vi "Dashboard Main.vi"() -> ()   [LabVIEW 2016]
uses:
  <vilib>/Utility/miscctls.llb/LVRowAndColumnTypeDef.ctl
  <vilib>/event_ctls.llb/eventvkey.ctl
  <vilib>/Rock Robotics/Network Tables/NT Read Numeric Array.vi
  <vilib>/Rock Robotics/Network Tables/NT Read Boolean.vi
  <vilib>/Rock Robotics/WPI/Dashboard/WPI_DashboardLogging Global.vi
  <vilib>/Math Plots/2D Math Plots/2D Compass/2D Compass Datatype/Public/Plot Helper (Vector).vi
  <vilib>/Math Plots/2D Math Plots/2D Compass/2D Compass Datatype/2D Compass Datatype.lvclass
panel:
  in  "Camera Settings Right":T1={"Frame Rate"=30, "Compression"=30, "Size"=1, "DB Camera Config"=FALSE} {"Frame Rate" scale=1.0..30.0; "Compression" scale=100.0..-1.0; "Size" items=["640x480", "320x240", "160x120"]}
  in  "Camera Name Right":string(combo)="No Camera Selection"
  out "Camera Info":cluster{"Mbps LED":bool, "Mbps":dbl, "fps":dbl} {"fps" format="%#.1g"; "Mbps" format="%#.1g"}
  in  "Camera Settings":T1={"Frame Rate"=30, "Compression"=30, "Size"=1, "DB Camera Config"=FALSE} {"Frame Rate" scale=1.0..30.0; "Compression" scale=100.0..-1.0; "Size" items=["640x480", "320x240", "160x120"]}
  in  "TCP":refnum<k5>
  in  "Rec Mode":enum32{"Stop", "Record", "Playback"}(radio)
  out "Robot IP":string
  out "Image Message":string="Timeout in Camera Communications"
  in  "Dashboard Tab":T2(tab)
  in  "Select Auto":string(combo)="Select Autonomous ..."
  out "NT Connection":bool
  out "MotorChart R":cluster{"Numeric":dbl, "Numeric":dbl}(graph)
  out "MotorChart L":cluster{"Numeric":dbl, "Numeric":dbl}(graph)
  out "MotorSliders R":cluster{"MotorSlide1":dbl, "MotorSlide2":dbl} {"MotorSlide2" scale=-1.0..1.0 scale format="%#_2e"; "MotorSlide1" scale=-1.0..1.0 scale format="%#_2e"}
  out "MotorSliders L":cluster{"MotorSlide1":dbl, "MotorSlide2":dbl} {"MotorSlide2" scale=-1.0..1.0 scale format="%#_2e"; "MotorSlide1" scale=-1.0..1.0 scale format="%#_2e"}
  out "Gyro":dbl(knob) scale=0.0..360.0
  out "JS1 Z":dbl(slide) scale=-1.0..1.0 scale format="%#_2e"
  out "JS1 Graph":cluster{"X":dbl, "Y":dbl}[](graph)
  out "JS1 Buttons":T3
  out "JS2 Z":dbl(slide) scale=-1.0..1.0 scale format="%#_2e"
  out "JS2 Graph":cluster{"X":dbl, "Y":dbl}[](graph)
  out "JS2 Buttons":T3
  out "Mode":T4(ring)=enum."Auto Disabled"
  out "Camera Image Right":T5(plugin-control)
  in  "DB/String 9":string
  in  "DB/String 8":string
  in  "DB/String 7":string
  in  "DB/String 6":string
  in  "DB/String 5":string
  in  "DB/String 4":string
  in  "DB/String 3":string
  in  "DB/String 2":string
  in  "DB/String 1":string
  in  "DB/String 0":string
  in  "DB/Slider 0":dbl(slide) scale=0.0..5.0
  in  "DB/Slider 1":dbl(slide) scale=0.0..5.0
  in  "DB/Slider 2":dbl(slide) scale=0.0..5.0
  in  "DB/Slider 3":dbl(slide) scale=0.0..5.0
  out "DB/LED 3":bool
  out "DB/LED 2":bool
  out "DB/LED 1":bool
  out "DB/LED 0":bool
  in  "DB/Button 3":bool
  in  "DB/Button 2":bool
  in  "DB/Button 1":bool
  in  "DB/Button 0":bool caption="New Name"
  out "Position Z":dbl
  out "Position Y":dbl
  out "Position X":dbl
  out "Velocity Z":dbl
  out "Velocity Y":dbl
  out "Velocity X":dbl
  in  "Auto Select":dbl
  out "Horizontal Heading":u8(slide) scale=0.0..100.0
  out "Vertical Heading":u8(slide) scale=0.0..100.0
  out "Slow":bool
  out "Fast":bool
  out "Reversed":bool
  out "Right Speed":dbl(knob) scale=0.0..1.0
  out "Left Speed":dbl(knob) scale=0.0..1.0
  out "Right Encoder":dbl
  out "Left Encoder":dbl
  in  "Test Slider":dbl(slide) scale=0.0..100.0 scale format="%#_3g"
  in  "On/Off":bool caption="Solenoid"
  in  "Test Name":u16(ring) items=["Select the test to run..."]
  in  "Test Tree":string(tree)
  in  "Motor":cluster{"Value":dbl, "Enable":bool} {"Value" scale=-1.0..1.0 scale format="%#_3g"}
  out "Progress":T6 {"Test Progress" scale=0.0..100.0}
  in  "Rev/Fwd":cluster{"Forward":bool, "Reverse":bool}
  in  "Test Ring":u16(ring) items=["Monochrome", "Color"]
  out "Cmd Status":string
  in  "Execute Command":bool
  in  "Command Params":string[][](table)
  in  "Command Selection":i32(listbox)
  in  "CheckList":i32(listbox)
  out "Tree":string(tree)
  out "Camera Image":T5(plugin-control)
  out "Background":bool
  in  "Camera Name":string(combo)="No Camera Selection"
  # "HW"
  # "HW"
  # "Joysticks"
  # "Drive Motors"
  # "Front"
  # "Right"
  # "Left"
  # "Back"
  # "1. Center Auto\n2. Left Auto\n3. Right Auto\n\n** Defaults to 1"
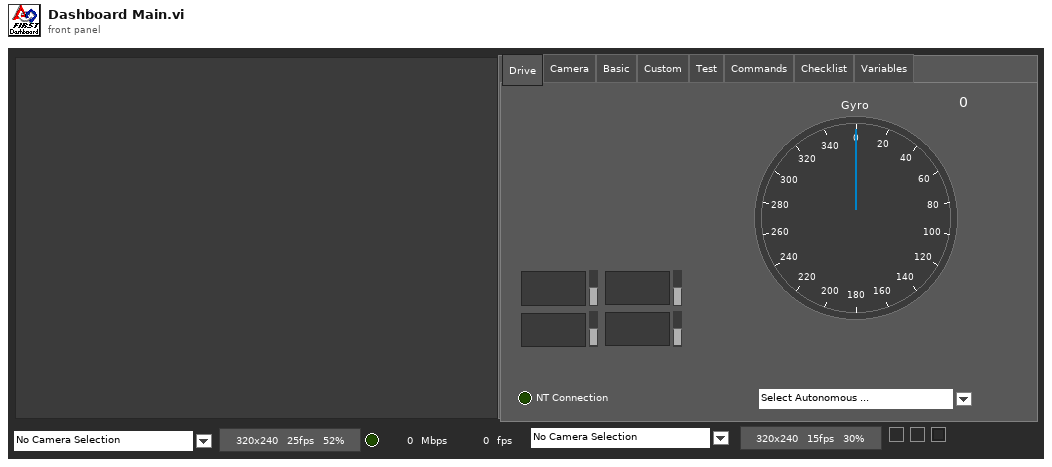
[diagram p1: front panel]
types:
  T1 = cluster{"Frame Rate":i32, "Compression":i32, "Size":u16, "DB Camera Config":bool}
  T2 = enum32{"Drive", "Camera", "Basic", "Custom", "Test", "Commands", "Checklist", "Variables"}
  T3 = cluster{bool, bool, bool, bool, bool, bool, bool, bool, bool, bool, bool, bool}
  T4 = enum8{"Tele-Op Disabled", "Tele-Op Enabled", "Auto Disabled", "Auto Enabled", "Test Disabled", "Test Enabled", "Disconnected", "No Code", "E-Stop"}
  T5 = typedef "IMAQ Image.ctl" = refnum<image>
  T6 = cluster{"Test Progress":u8, "Test Progress Text":string}
  T7 = typedef "Image Type" = u32
  T8 = cluster{"IDs":cluster{"RPC field ID":u16, "Unique ID":u16}, "String":string}
  T9 = enum32{"Drive", "Basic", "Custom", "Test", "Checklist", "Variables"}
  T10 = cluster{"Error Strings":string, "Disable Counts":cluster{u16, u16}, "Rail Faults":cluster{u16, u16, u16}, "Robot IP":string, "DB Mode":u8, "Event Info":cluster{"Name":string, "Type":u8, "Number":u16, "Replay":u8}}
  T11 = cluster{"Storage":cluster{"Disk Free":u64, "RAM Block":u32, "RAM free":u32}, "CPU Utilization":cluster{"CPU % ISR":sgl, "CPU % Time Crit":sgl, "CPU % Timed Str":sgl, "CPU % High":sgl, "CPU % Above":sgl, "CPU % Normal":sgl, "CPU % Low":sgl}, "CAN":cluster{"% Bus Utilization":sgl, "Bus Off Cnt":u32, "TX_FIFO Full Cnt":u32, "Receive Error Cnt":u8, "Transmit Error Cnt":u8}, "HID":cluster{"HID Outputs":u32, "Rumble Low":u16, "Rumble High":u16}[]}
  T12 = cluster{"Status bits":cluster{"Test Mode":bool, "Autonomous":bool, "Enabled":bool, "Code Start":bool, "Brownout":bool, "Reserved 2":bool, "Reserved 3":bool, "E-Stop":bool}, "Code Trace":cluster{"Disabled":bool, "TeleOp":bool, "Auto":bool, "Test":bool}, "Controller Type":enum16{"unknown", "cRIO", "roboRio"}, "Code?":enum16{"unknown", "noCode", "code"}, "Battery V":dbl}
  T13 = cluster{"Control Bits":cluster{"TestMode":bool, "Autonomous":bool, "Enabled":bool, "FMS Present":bool, bool, bool, bool, "E-Stop":bool}, "Team Station ":u8, "Countdown":sgl, "Joystick Values":cluster{"Axes":dbl[], "Buttons":bool[], "POVs":i16[]}[]}
  T14 = cluster{"Axes":dbl[], "Buttons":bool[], "POVs":i16[]}[]
  T15 = cluster{"Axes":dbl[], "Buttons":bool[], "POVs":i16[]}
  T16 = cluster{"Buttons[0]":bool, "Buttons[1]":bool, "Buttons[2]":bool, "Buttons[3]":bool, "Buttons[4]":bool, "Buttons[5]":bool, "Buttons[6]":bool, "Buttons[7]":bool, "Buttons[8]":bool, "Buttons[9]":bool, "Buttons[10]":bool, "Buttons[11]":bool}
  T17 = cluster{"Camera Image":refnum<vi>, "Dashboard Tab":refnum<vi>, "Background":refnum<vi>, "Rec Mode":refnum<vi>, "Test Slider":refnum<vi>, "On/Off ":refnum<vi>, "Test Ring":refnum<vi>, "Rev/Fwd":refnum<vi>, "Test Name":refnum<vi>, "Motor":refnum<vi>, "Progress":refnum<vi>, "CheckList":refnum<vi>, "Tree":refnum<vi>, "Test Tree":refnum<vi>, "Command Params":refnum<vi>, "Command Selection":refnum<vi>, "Execute Command":refnum<vi>, "Cmd Status":refnum<vi>, "Camera Settings":refnum<vi>, "Camera Name":refnum<vi>, "Camera Info":refnum<vi>, "Camera Settings Right":refnum<vi>, "Camera Name Right":refnum<vi>, "Camera Image Right":refnum<vi>}
  T18 = cluster{"Operation":enum16{"Update", "Clear"}, "Color Box":u32}[]
  T19 = typedef "eventvkey.ctl" = enum16{"ASCII", "Enter", "Return", "Shift", "Ctrl", "Alt", "Cmd", "Opt", "Caps", "NumLock", "Clear", "Break", "Up", "Down", "Left", "Right", "Insert", "Delete", "Home", "End", "PageUp", "PageDown", "Escape", "Help", "Pause", "ScrollLock", "F1", "F2", "F3", "F4", "F5", "F6", "F7", "F8", "F9", "F10", "F11", "F12", "F13", "F14", "F15", "F16", "F17", "F18", "F19", "F20", "F21", "F22", "F23", "F24", "Play", "VolumeUp", "VolumeDown", "Mute", "Two Byte Char"}
  T20 = cluster{"Image Size":bool, "Image Type":bool, "Pixel Value":bool, "ROI Information":bool, "Zoom Factor":bool}
  T21 = cluster{"Operation":enum16{"Update", "Clear"}, "Color Box":u32}
  T22 = typedef "LVRowAndColumnTypeDef.ctl" = cluster{"Row":i32, "Column":i32}
  T23 = cluster{"Shift":bool, "Ctrl":bool, "Alt":bool, "Cmd":bool, "Opt":bool}
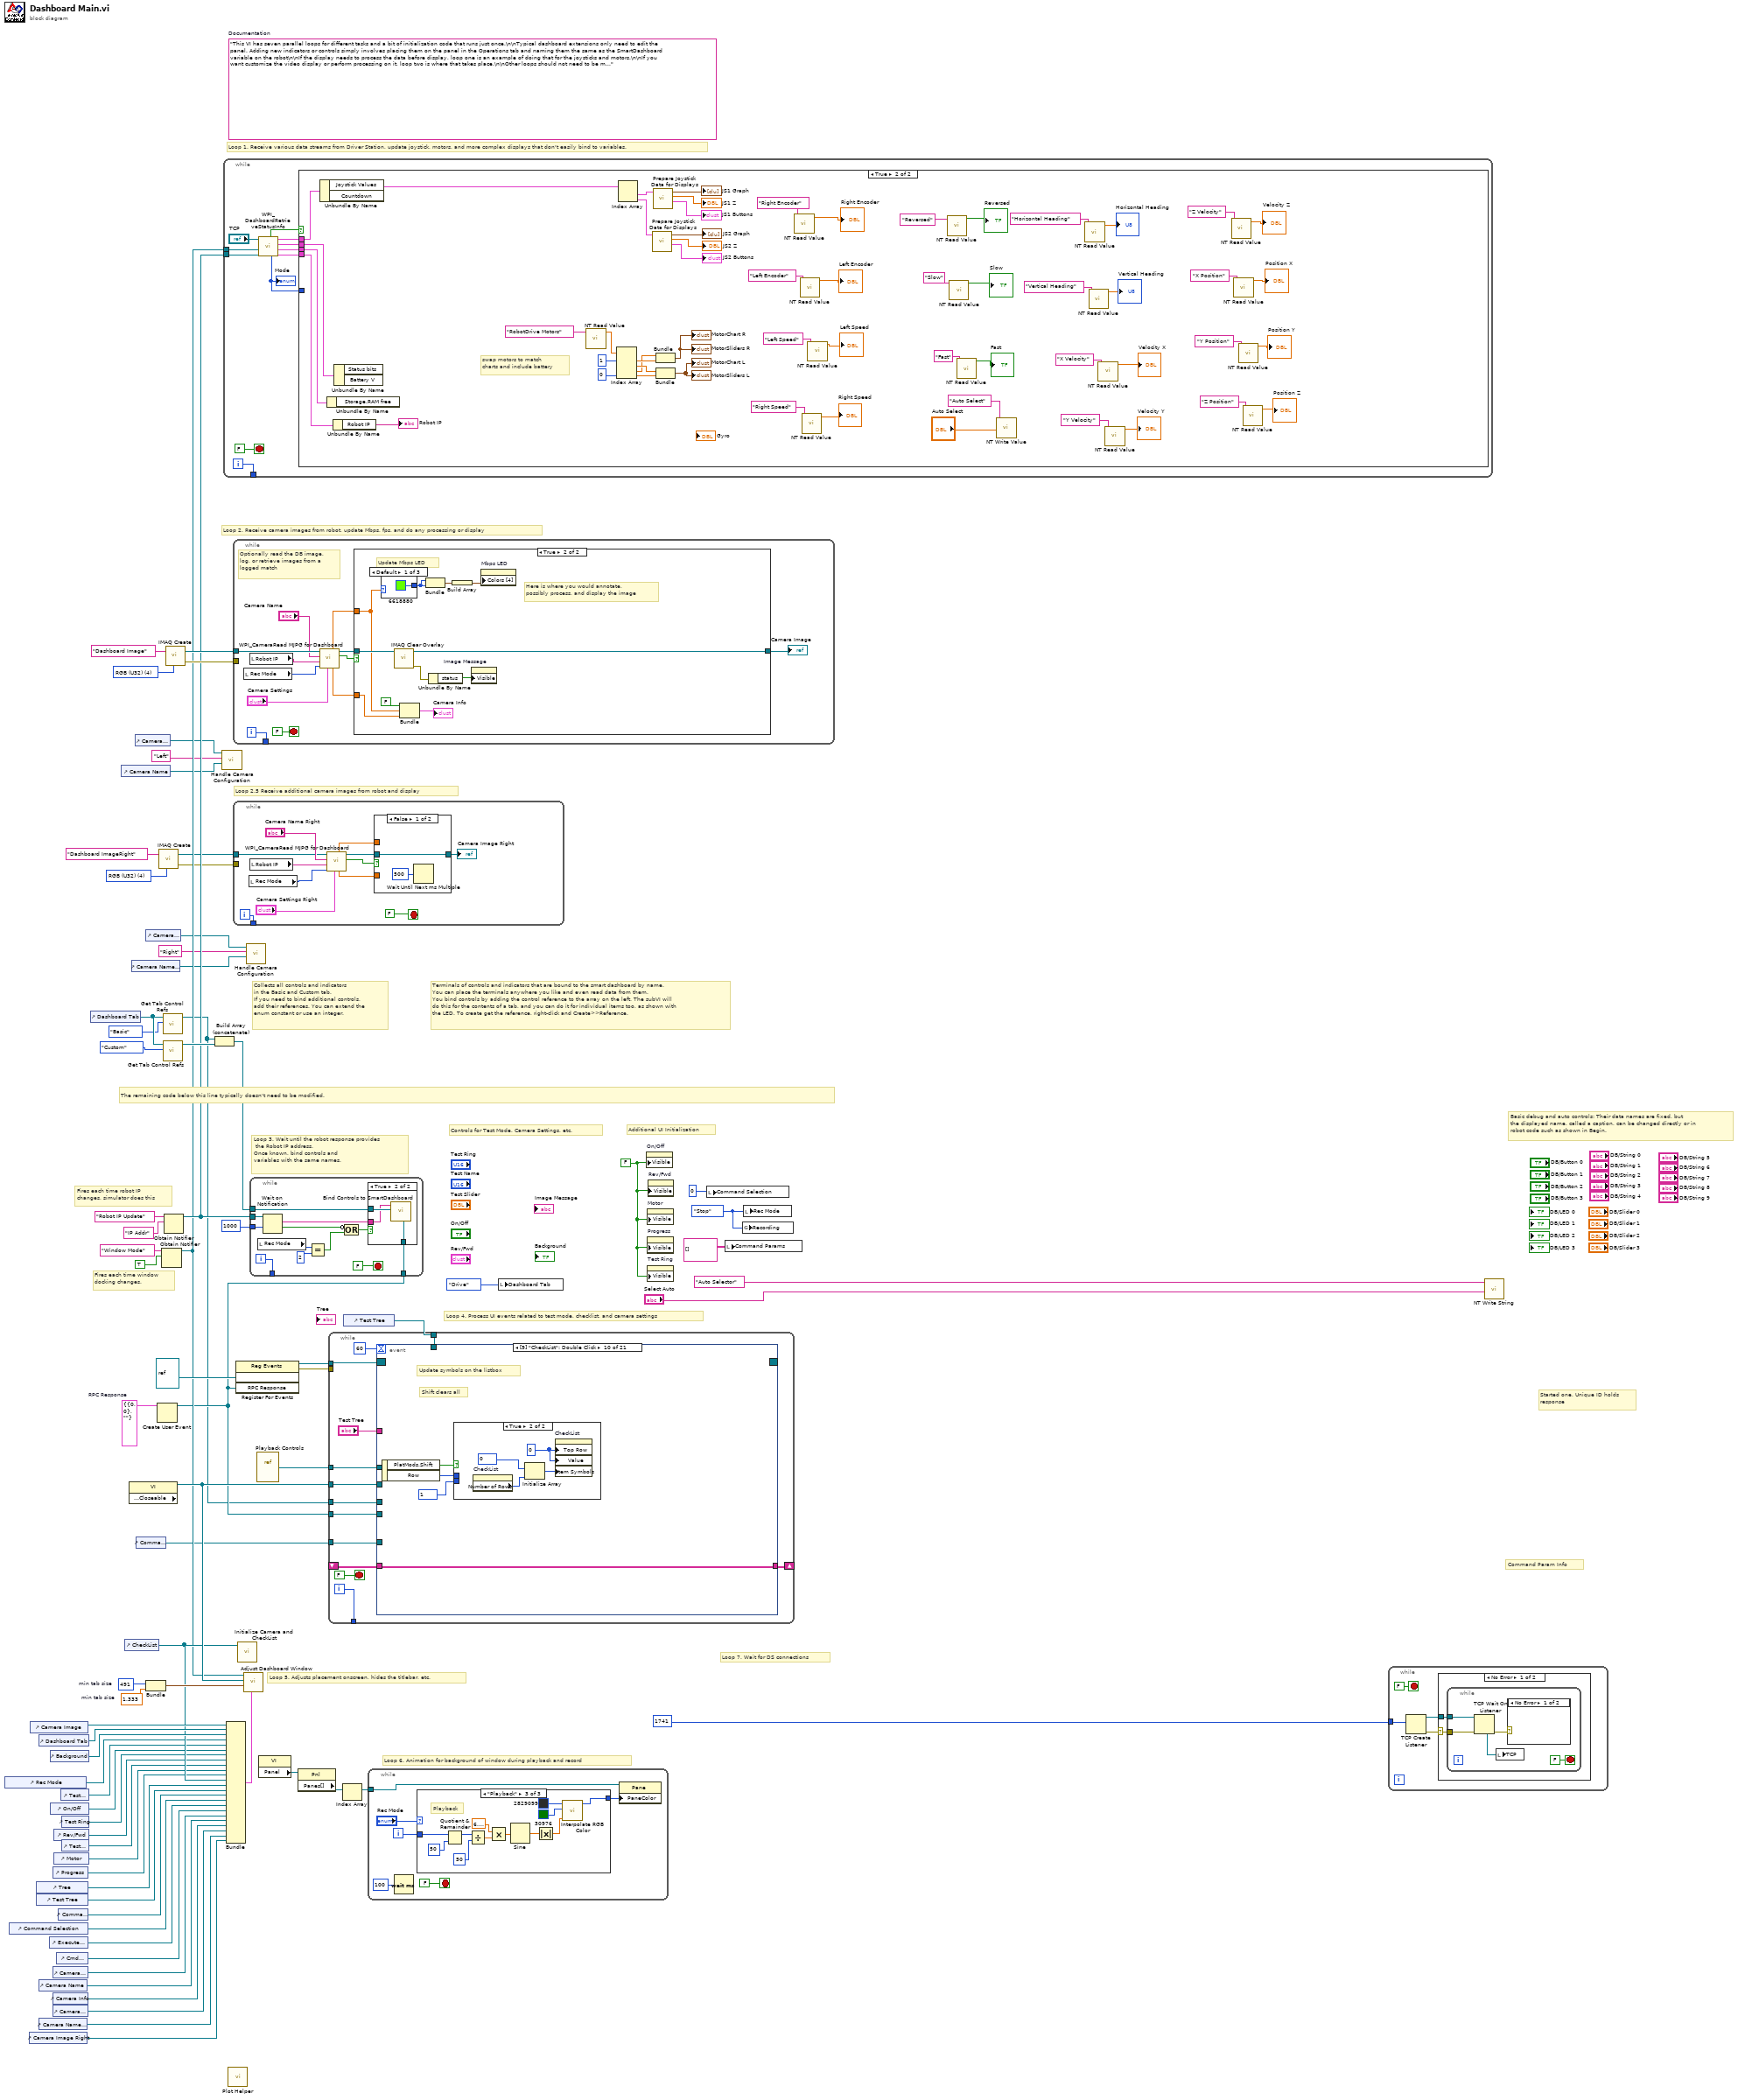
[diagram p0: block diagram]
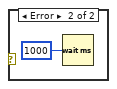
[diagram p3: hidden frame]
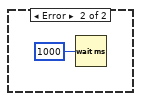
[diagram p4: hidden frame]
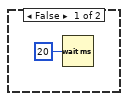
[diagram p5: hidden frame]
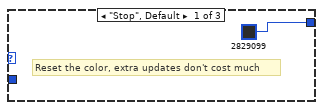
[diagram p6: hidden frame]
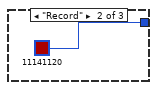
[diagram p7: hidden frame]
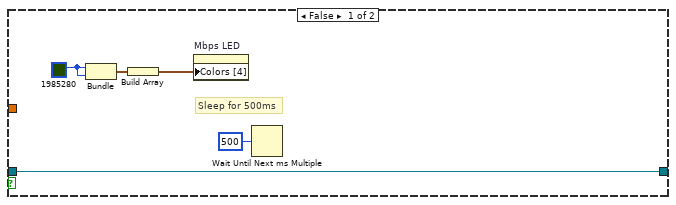
[diagram p9: hidden frame]
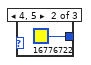
[diagram p10: hidden frame]
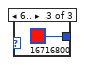
[diagram p11: hidden frame]
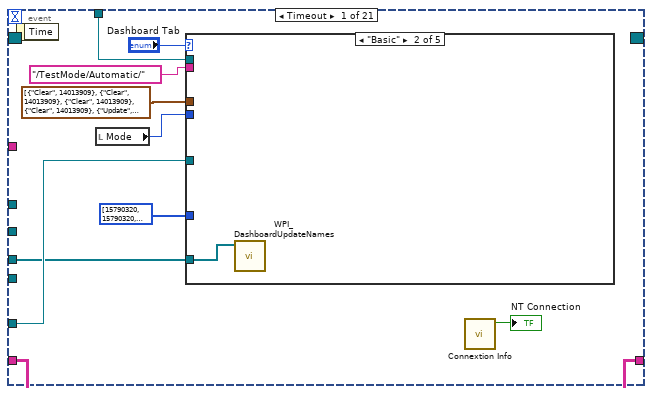
[diagram p12: hidden frame]
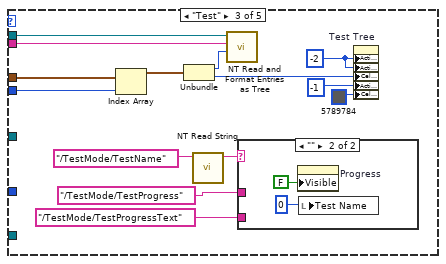
[diagram p14: hidden frame]
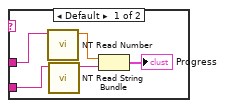
[diagram p15: hidden frame]
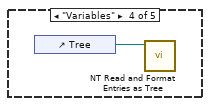
[diagram p16: hidden frame]
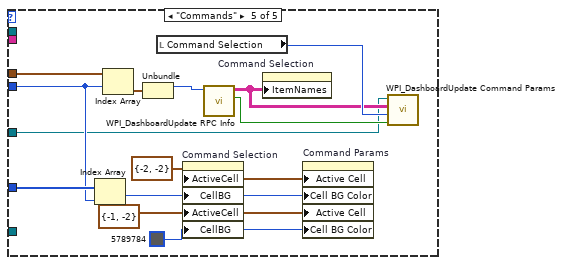
[diagram p17: hidden frame]
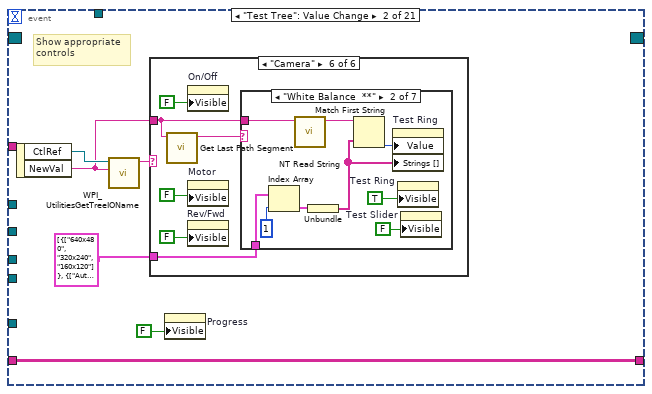
[diagram p18: hidden frame]
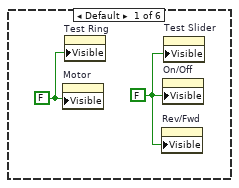
[diagram p19: hidden frame]
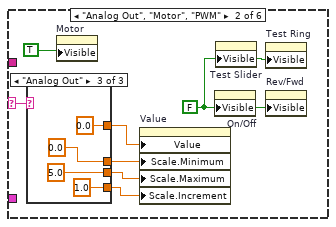
[diagram p20: hidden frame]
diagram:
  w10 = T7 4 items=["Grayscale (U8)", "Grayscale (I16)", "Grayscale (SGL)", "Complex (CSG)", "RGB (U32)", "HSL (U32)", "RGB (U64)"] ("Image Type")
  w26 = T8 {"IDs"={"RPC field ID"=0, "Unique ID"=0}, "String"=""}  # RPC Response
  w51 = 491  # min tab size
  w50 = 1.333  # min tab size
  w58 = enum32{"Stop", "Record", "Playback"}."Stop" ("Rec Mode")
  w33 = FALSE ("Visible")
  (unwired) "This VI has seven parallel loops for different tasks and a bit of initialization code that runs just once.\n\nTypical dashboard extensions only need to edit the panel. Adding new indicators or controls simply involves placing them on the panel in the Operations tab and naming them the same as the SmartDashboard variable on the robot\n\nIf the display needs to process the data before display, loop one is an example of doing that for the joysticks and motors.\n\nIf you want customize the video display or perform processing on it, loop two is where that takes place.\n\nOther loops should not need to be modified. They are pretty standard, and document the task they perform."  # Documentation
  w75 = T7 4 items=["Grayscale (U8)", "Grayscale (I16)", "Grayscale (SGL)", "Complex (CSG)", "RGB (U32)", "HSL (U32)", "RGB (U64)"] ("Image Type")
  # "Loop 2.5 Receive additional camera images from robot and display"
  # "Command Param Info"
  # "Started one, Unique ID holds\nresponse"
  # "Loop 7. Wait for DS connections"
  # "Basic debug and auto controls: Their data names are fixed, but\nthe displayed name, called a caption, can be changed directly or in\nrobot code such as shown in Begin."
  # "Controls for Test Mode, Camera Settings, etc."
  # "Additional UI Initialization"
  # "Loop 6. Animation for background of window during playback and record"
  # "Fires each time robot IP\nchanges, simulator does this"
  # "Fires each time window\ndocking changes."
  # "Collects all controls and indicators\nin the Basic and Custom tab.\nIf you need to bind additional controls,\nadd their references. You can extend the\nenum constant or use an integer."
  # "The remaining code below this line typically doesn't need to be modified."
  # "Loop 4. Process UI events related to test mode, checklist, and camera settings"
  # "Terminals of controls and indicators that are bound to the smart dashboard by name.\nYou can place the terminals anywhere you like and even read data from them.\nYou bind controls by adding the control reference to the array on the left. The subVI will\ndo this for the contents of a tab, and you can do it for individual items too, as shown with\nthe LED. To create get the reference, right-click and Create>>Reference."
  # "Loop 3. Wait until the robot response provides\n the Robot IP address.\nOnce known, bind controls and\nvariables with the same names."
  # "Loop 5. Adjusts placement onscreen, hides the titlebar, etc."
  # "Loop 1. Receive various data streams from Driver Station, update joystick, motors, and more complex displays that don't easily bind to variables."
  # "Loop 2. Receive camera images from robot, update Mbps, fps, and do any processing or display"
  n1 = control-ref of="Rec Mode"() -> (w39:refnum<vi>)
  n2 = control-ref of="Command Selection"() -> (w25:refnum<vi>)
  n3 = control-ref of="Camera Image Right"() -> (w1:refnum<vi>)
  n4 = control-ref of="Camera Image"() -> (w53:refnum<vi>)
  n5 = control-ref of="Tree"() -> (w43:refnum<vi>)
  n6 = control-ref of="Test Tree"() -> (w42:refnum<vi>)
  n7 = control-ref of="Dashboard Tab"() -> (w52:refnum<vi>)
  n8 = control-ref of="Camera Name"() -> (w16:refnum<vi>)
  n9 = control-ref of="Camera Name Right"() -> (w2:refnum<vi>)
  n10 = control-ref of="Execute Command"() -> (w27:refnum<vi>)
  n11 = control-ref of="Background"() -> (w48:refnum<vi>)
  n12 = control-ref of="On/Off"() -> (w37:refnum<vi>)
  n13 = control-ref of="Progress"() -> (w34:refnum<vi>)
  n14 = control-ref of="Camera Settings"() -> (w17:refnum<vi>)
  n15 = control-ref of="Camera Info"() -> (w15:refnum<vi>)
  n16 = control-ref of="Camera Settings Right"() -> (w3:refnum<vi>)
  n17 = control-ref of="Rev/Fwd"() -> (w35:refnum<vi>)
  n18 = control-ref of="Motor"() -> (w40:refnum<vi>)
  n19 = control-ref of="Cmd Status"() -> (w21:refnum<vi>)
  n20 = control-ref of="Command Params"() -> (w28:refnum<vi>)
  n21 = control-ref of="Test Slider"() -> (w38:refnum<vi>)
  n22 = control-ref of="Test Ring"() -> (w36:refnum<vi>)
  n23 = control-ref of="Test Name"() -> (w41:refnum<vi>)
  n24 = control-ref of="Dashboard Tab"() -> (w56:refnum<vi>)
  n25 = control-ref of="Camera Name"() -> (w18:refnum<vi>)
  n26 = control-ref of="CheckList"() -> (w44:refnum<vi>)
  n27 = property class="VI" props=["Front Panel.Closeable"]() -> (reference out=w57:refnum<vi>)  [unwired: 2 in, 2 out]
  n28 = control-ref of="Camera Name Right"() -> (w6:refnum<vi>)
  n29 = control-ref of="Camera Settings"() -> (w19:refnum<vi>)
  n30 = control-ref of="Command Params"() -> (w20:refnum<vi>)
  n31 = control-ref of="Camera Settings Right"() -> (w7:refnum<vi>)
  n32 = Bundle("min tab size"=w51, "min tab size"=w50) -> (w49:cluster{"min tab size":i32, "min tab size":dbl})  [unwired: 1 in]
  n33 = Create User Event(user event datatype=w26) -> (user event=w22:refnum<user-event>)  [unwired: 1 in, 1 out]
  n34 = call "IMAQ Create"("Image Name"="Dashboard ImageRight", "Image Type"=w10) -> ("New Image"=w9:T5, "error out"=w8:errorcluster)  [unwired: 2 in, 1 out]
  n35 = Obtain Notifier(name (unnamed)="Window Mode", notification data type=TRUE) -> (notifier out=w31:refnum<notifier>)  [unwired: 2 in, 2 out]
  n36 = call <vilib>:"Get Tab Control Refs.vi"("Page Index"=T9."Basic" ("Dashboard Tab"), "TabControl in"=w56) -> ("ControlsOnPage"=w14:refnum<vi>[])  [unwired: 9 in]
  n37 = call <vilib>:"Get Tab Control Refs.vi"("Page Index"=T9."Custom" ("Dashboard Tab"), "TabControl in"=w56) -> ("ControlsOnPage"=w55:refnum<vi>[])  [unwired: 9 in]
  n38 = Obtain Notifier(name (unnamed)="Robot IP Update", notification data type="IP Addr" ("name (unnamed)")) -> (notifier out=w32:refnum<notifier>)  [unwired: 2 in, 2 out]
  n39 = call "IMAQ Create"("Image Name"="Dashboard Image", "Image Type"=w75) -> ("New Image"=w73:T5, "error out"=w72:errorcluster)  [unwired: 2 in, 1 out]
  n40 = Build Array (concatenate)(w14, w55) -> (w54:refnum<vi>[])
  n41 = call "Handle Camera Configuration.vi"("CameraNameRef"=w18, "Camera File Name"="Left", "ClusterRef"=w19) -> ()  [unwired: 9 in]
  n42 = while {
    tunnel: [w85] -> _
    tunnel: w32 -> [w79]
    tunnel: w31 -> [w76]
    i -> [w85]
    stop <- FALSE stop-if-true
    n43 = call <vilib>:"WPI_DashboardRetrieveStatusInfo.vi"("Binding Refnum"=w79, "Window Mode Notifier"=w76, "TCP Cnx"="TCP") -> ("Power and Errors"=w80:T10, "Robot Metrics"=w83:T11, "Status Info"=w84:T12, "Control Info"=w81:T13, "Robot Mode"=w78:T4, "Process?"=w82:bool)  [unwired: 3 in]
    "Mode" <- w78
    n44 = case shown="True" w82 {
      tunnel: w84 -> [_ w143]
      tunnel: w83 -> [_ w142]
      tunnel: w81 -> [_ w141]
      tunnel: w80 -> [_ w140]
      tunnel: w78 -> [_ _]
      frame False {
        n45 = Wait (ms)(milliseconds to wait=u32 20) -> ()  [unwired: 1 out]
      }
      frame True {
        # "swap motors to match\ncharts and include battery"
        n46 = Unbundle By Name(w141) -> ("Joystick Values"=w131:T14)  [unwired: 1 out]
        n47 = Unbundle By Name(w142) -> ()  [unwired: 1 out]
        n48 = Unbundle By Name(w140) -> ("Robot IP"=→"Robot IP":string)
        n49 = Unbundle By Name(w143) -> ()  [unwired: 2 out]
        n50 = call-poly <vilib>:"NT Read Value.vi"("Name"="RobotDrive Motors") -> ("Numeric Array"=w121:dbl[])  [unwired: 9 in, 1 out]
        n51 = Index Array(array=w121, index #1=1, index #4=0) -> (element #1=w135:dbl, element #2=w136:dbl, element #3=w134:dbl, element #4=w139:dbl)  [unwired: 2 in]
        n52 = Index Array(array=w131) -> (element #1=w130:T15, element #2=w126:T15)  [unwired: 2 in]
        n53 = call "Prepare Joystick Data for Displays.vi"("Joystick Values"=w126) -> ("Buttons"=→"JS2 Buttons":T16, "Z Axis"=→"JS2 Z":dbl, "Cartesian Data"=→"JS2 Graph":cluster{"X axis":dbl, "X axis":dbl}[])  [unwired: 8 in]
        n54 = call "Prepare Joystick Data for Displays.vi"("Joystick Values"=w130) -> ("Buttons"=→"JS1 Buttons":T16, "Z Axis"=→"JS1 Z":dbl, "Cartesian Data"=→"JS1 Graph":cluster{"X axis":dbl, "X axis":dbl}[])  [unwired: 8 in]
        n55 = Bundle("Numeric"=w134, "Numeric"=w135) -> (→"MotorChart R" →"MotorSliders R":cluster{"Numeric":dbl, "Numeric":dbl})  [unwired: 1 in]
        n56 = Bundle("Numeric"=w136, "Numeric"=w139) -> (→"MotorChart L" →"MotorSliders L":cluster{"Numeric":dbl, "Numeric":dbl})  [unwired: 1 in]
        n57 = call-poly <vilib>:"NT Read Value.vi"("Name"="Right Encoder") -> ("Numeric"=→"Right Encoder":dbl)  [unwired: 9 in, 1 out]
        n58 = call-poly <vilib>:"NT Read Value.vi"("Name"="Left Encoder") -> ("Numeric"=→"Left Encoder":dbl)  [unwired: 9 in, 1 out]
        n59 = call-poly <vilib>:"NT Read Value.vi"("Name"="Right Speed") -> ("Numeric"=→"Right Speed":dbl)  [unwired: 9 in, 1 out]
        n60 = call-poly <vilib>:"NT Read Value.vi"("Name"="Left Speed") -> ("Numeric"=→"Left Speed":dbl)  [unwired: 9 in, 1 out]
        n61 = call-poly <vilib>:"NT Read Value.vi"("Name"="Reversed") -> ("Boolean"=→"Reversed":bool)  [unwired: 9 in, 1 out]
        n62 = call-poly <vilib>:"NT Read Value.vi"("Name"="Slow") -> ("Boolean"=→"Slow":bool)  [unwired: 9 in, 1 out]
        n63 = call-poly <vilib>:"NT Read Value.vi"("Name"="Fast") -> ("Boolean"=→"Fast":bool)  [unwired: 9 in, 1 out]
        n64 = call-poly <vilib>:"NT Write Value.vi"("Numeric"="Auto Select", "Name"="Auto Select") -> ()  [unwired: 9 in, 1 out]
        n65 = call-poly <vilib>:"NT Read Value.vi"("Name"="Horizontal Heading") -> ("Numeric"=→"Horizontal Heading":dbl)  [unwired: 9 in, 1 out]
        n66 = call-poly <vilib>:"NT Read Value.vi"("Name"="Vertical Heading") -> ("Numeric"=→"Vertical Heading":dbl)  [unwired: 9 in, 1 out]
        n67 = call-poly <vilib>:"NT Read Value.vi"("Name"="X Velocity") -> ("Numeric"=→"Velocity X":dbl)  [unwired: 9 in, 1 out]
        n68 = call-poly <vilib>:"NT Read Value.vi"("Name"="Y Velocity") -> ("Numeric"=→"Velocity Y":dbl)  [unwired: 9 in, 1 out]
        n69 = call-poly <vilib>:"NT Read Value.vi"("Name"="Z Velocity") -> ("Numeric"=→"Velocity Z":dbl)  [unwired: 9 in, 1 out]
        n70 = call-poly <vilib>:"NT Read Value.vi"("Name"="X Position") -> ("Numeric"=→"Position X":dbl)  [unwired: 9 in, 1 out]
        n71 = call-poly <vilib>:"NT Read Value.vi"("Name"="Y Position") -> ("Numeric"=→"Position Y":dbl)  [unwired: 9 in, 1 out]
        n72 = call-poly <vilib>:"NT Read Value.vi"("Name"="Z Position") -> ("Numeric"=→"Position Z":dbl)  [unwired: 9 in, 1 out]
      }
    }
  }
  n73 = Bundle("Camera Image"=w53, "Dashboard Tab"=w52, "Background"=w48, "Rec Mode"=w39, "Test Slider"=w38, "On/Off"=w37, "Test Ring"=w36, "Rev/Fwd"=w35, "Test Name"=w41, "Motor"=w40, "Progress"=w34, "CheckList"=w44, "Tree"=w43, "Test Tree"=w42, "Command Params"=w28, "Command Selection"=w25, "Execute Command"=w27, "Cmd Status"=w21, "Camera Settings"=w17, "Camera Name"=w16, "Camera Info"=w15, "Camera Settings Right"=w3, "Camera Name Right"=w2, "Camera Image Right"=w1) -> (w45:T17)  [unwired: 1 in]
  n74 = call-poly <vilib>:"Plot Helper.vi"() -> ()  [unwired: 4 in, 8 out]
  n75 = while {
    tunnel: w73 -> [w153]
    tunnel: w72 -> [_]
    tunnel: [w154] -> _
    i -> [w154]
    stop <- FALSE stop-if-true
    # "Optionally read the DB image,\nlog, or retrieve images from a\nlogged match"
    n76 = local read "Rec Mode"() -> (w149:enum32{"Stop", "Record", "Playback"})
    n77 = local read "Robot IP"() -> (w148:string)
    n78 = call <vilib>:"WPI_CameraRead MJPG for Dashboard.vi"("Camera Settings"="Camera Settings", "Rec Mode"=w149, "Robot IP"=w148, "Camera Name"="Camera Name", "Refnum in"=w153) -> ("Active"=w151:bool, "Refnum out"=w152:T5, "FPS"=w150:dbl, "Bandwidth (Mbps)"=w147:dbl)  [unwired: 3 in]
    n79 = case shown="True" w151 {
      tunnel: w152 -> [w156 w167]
      tunnel: w147 -> [_ w164]
      tunnel: w150 -> [_ w165]
      tunnel: [w156 w161] -> w144
      frame False {
        w158 = u32 1985280 ("Color Box")
        # "Sleep for 500ms"
        n80 = Bundle("Color Box"=w158, "Color Box"=w158) -> (w159:cluster{"Color Box":u32, "Color Box":u32})  [unwired: 1 out]
        n81 = Build Array(w159) -> (w157:cluster{"Color Box":u32, "Color Box":u32}[])
        n82 = property on="Mbps LED" class="Bool (strict)"("Colors [4]"=w157) -> ()  [unwired: 2 in, 2 out]
        n83 = Wait Until Next ms Multiple(millisecond multiple=u32 500) -> ()  [unwired: 1 out]
      }
      frame True {
        # "Here is where you would annotate,\npossibly process, and display the image"
        # "Update Mbps LED"
        n84 = case shown="Default" w164 {
          tunnel: [u32 6618880 ("Color Box") u32 16776722 ("Color Box") u32 16716800 ("Color Box")] -> w168
          frame Default {
          }
          frame 4, 5 {
          }
          frame 6.. {
          }
        }
        n85 = call "IMAQ Clear Overlay"("Image"=w167) -> ("error out"=w170:errorcluster, "Image Out"=w161:T5)  [unwired: 2 in, 7 out]
        n86 = Bundle(FALSE, "Bandwidth (Mbps)"=w164, "FPS"=w165) -> (→"Camera Info":cluster{bool, "Bandwidth (Mbps)":dbl, "FPS":dbl})  [unwired: 1 in]
        n87 = Bundle("Color Box"=w168, "Color Box"=w168) -> (w169:cluster{"Color Box":u32, "Color Box":u32})  [unwired: 1 out]
        n88 = Unbundle By Name(w170) -> ("status"=w171:bool)
        n89 = Build Array(w169) -> (w166:cluster{"Color Box":u32, "Color Box":u32}[])
        n90 = property on="Image Message" class="Str"("Visible"=w171) -> ()  [unwired: 2 in, 2 out]
        n91 = property on="Mbps LED" class="Bool (strict)"("Colors [4]"=w166) -> ()  [unwired: 2 in, 2 out]
      }
    }
    "Camera Image" <- w144
  }
  n92 = while {
    tunnel: w9 -> [w185]
    tunnel: w8 -> [_]
    tunnel: [w179] -> _
    i -> [w179]
    stop <- FALSE stop-if-true
    n93 = local read "Rec Mode"() -> (w183:enum32{"Stop", "Record", "Playback"})
    n94 = local read "Robot IP"() -> (w184:string)
    n95 = call <vilib>:"WPI_CameraRead MJPG for Dashboard.vi"("Camera Settings"="Camera Settings Right", "Rec Mode"=w183, "Robot IP"=w184, "Camera Name"="Camera Name Right", "Refnum in"=w185) -> ("Active"=w178:bool, "Refnum out"=w181:T5, "FPS"=w176:dbl, "Bandwidth (Mbps)"=w177:dbl)  [unwired: 3 in]
    n96 = case shown="False" w178 {
      tunnel: w181 -> [w187 w189]
      tunnel: w177 -> [_ _]
      tunnel: w176 -> [_ _]
      tunnel: [w187 w189] -> w175
      frame False {
        n97 = Wait Until Next ms Multiple(millisecond multiple=u32 500) -> ()  [unwired: 1 out]
      }
      frame True {
      }
    }
    "Camera Image Right" <- w175
  }
  n98 = register-events(refnum<vi> refnum, w22) -> (reference out=w62:refnum<event-registration>, error out=w61:errorcluster)  [unwired: 2 in]
  n99 = call "Initialize Camera and CheckList.vi"("ListBox in"=w44) -> ()  [unwired: 11 in]
  n100 = call "Adjust Dashboard Window.vi"("Sizing Refnums"=w45, "Size Constraints"=w49, "VI"=w57, "WIn Mode"=w31) -> ()  [unwired: 8 in]
  n101 = call "Handle Camera Configuration.vi"("CameraNameRef"=w6, "Camera File Name"="Right", "ClusterRef"=w7) -> ()  [unwired: 9 in]
  n102 = while {
    tunnel: w54 -> [w201]
    tunnel: w32 -> [w199]
    tunnel: [w197] -> _
    tunnel: u32 1000 ("milliseconds to wait") -> [w196]
    tunnel: w22 -> [w190]
    i -> [w197]
    stop <- FALSE stop-if-true
    n103 = local read "Rec Mode"() -> (w192:enum32{"Stop", "Record", "Playback"})
    n104 = Wait on Notification(notifier=w199, timeout in ms (-1)=w196) -> (notification=w198:string, timed out?=w194:bool)  [unwired: 2 in, 2 out]
    n105 = Equal?(x=w192, y=u16 2 ("Rec Mode")) -> (x = y?=w193:bool)
    n106 = Compound Arithmetic op=OR(invert w194, w193) -> (w195:bool)
    n107 = case shown="True" w195 {
      tunnel: w201 -> [_ w204]
      tunnel: w198 -> [_ w203]
      tunnel: w190 -> [_ w202]
      frame False {
      }
      frame True {
        n108 = call <vilib>:"Bind Controls to SmartDashboard.vi"("RPC ref"=w202, "Bound Control Refs"=w204, "Server IP Address"=w203) -> ()  [unwired: 9 in]
      }
    }
  }
  n109 = vi-ref "Playback Controls.vi"() -> (w63:refnum<vi>)
  n110 = property class="VI"() -> ("Panel"=w65:refnum<vi>)  [unwired: 2 in, 2 out]
  n111 = property class="Pnl"(reference=w65) -> ("Panes[]"=w66:refnum<vi>[])  [unwired: 1 in, 2 out]
  n112 = Index Array(array=w66) -> (element=w64:refnum<vi>)  [unwired: 1 in]
  n113 = control-ref of="Test Tree"() -> (w67:refnum<vi>)
  n114 = while {
    tunnel: [w214] -> _
    tunnel: w67 -> [w213]
    tunnel: w63 -> [w212]
    tunnel: w62 -> [w211]
    tunnel: w61 -> [_]
    tunnel: w57 -> [w210]
    tunnel: w22 -> [w209]
    tunnel: w20 -> [w208]
    shift-right: [w207] -> _
    shift-left: _ -> [w206]
    tunnel: w14 -> [w205]
    i -> [w214]
    stop <- FALSE stop-if-true
    n115 = event shown="[9] \"CheckList\": Double Click" {
      selector: w211 -> [_ _ _ _ _ _ _ _ _ _ _ _ _ _ _ _ _ _ _ _ _]
      dyn-events: [_ _ _ _ _ _ _ _ _ _ _ _ _ _ _ _ w470 _ _ _ _] -> _
      timeout: u32 60 ("milliseconds to wait") -> [_ _ _ _ _ _ _ _ _ _ _ _ _ _ _ _ _ _ _ _ _]
      tunnel: w213 -> [w226 _ _ _ _ _ _ _ _ _ _ _ _ _ _ _ _ _ _ _ _]
      tunnel: "Test Tree" -> [_ _ _ _ _ _ _ _ _ _ _ w437 w445 w447 w451 w459 _ _ _ _ _]
      tunnel: w212 -> [_ _ _ _ _ _ _ _ _ _ _ _ _ _ _ _ w472 _ w490 _ _]
      tunnel: w210 -> [_ _ _ _ _ _ _ _ _ _ _ _ _ _ _ _ w468 _ _ _ _]
      tunnel: w209 -> [_ _ _ _ _ _ _ _ _ _ _ _ _ _ _ _ w464 _ _ _ _]
      tunnel: w208 -> [w221 _ _ _ _ _ w388 _ _ _ _ _ _ _ _ _ _ _ _ _ _]
      tunnel: [w220 w265 w367 w372 w381 w385 w386 w395 w405 w412 w424 w436 w443 w446 w450 w458 w463 w485 w487 w491 w502] -> w207
      tunnel: w206 -> [w220 w265 w367 w372 w381 w385 w386 _ _ w412 w424 w436 w443 w446 w450 w458 w463 w485 w487 w491 w502]
      tunnel: w205 -> [w218 _ _ _ _ _ _ _ _ _ _ _ _ _ _ _ _ _ _ _ _]
      event Timeout {
        n116 = event-data() -> ()  [unwired: 1 in, 1 out]
        n117 = local read "Mode"() -> (w223:T4)
        n118 = case shown="\"Basic\"" "Dashboard Tab" {
          tunnel: w226 -> [_ _ w242 _ _]
          tunnel: "/TestMode/Automatic/" ("Name Pattern") -> [_ _ w241 _ _]
          tunnel: T18 [{"Operation"=enum."Clear", "Color Box"=14013909}, {"Operation"=enum."Clear", "Color Box"=14013909}, {"Operation"=enum."Clear", "Color Box"=14013909}, {"Operation"=enum."Clear", "Color Box"=14013909}, {"Operation"=enum."Update", "Color Box"=14013909}, {"Operation"=enum."Update", "Color Box"=16777215}, {"Operation"=enum."Clear", "Color Box"=14013909}, {"Operation"=enum."Clear", "Color Box"=14013909}, {"Operation"=enum."Clear", "Color Box"=14013909}] -> [_ _ w234 _ w258]
          tunnel: w223 -> [_ _ w233 _ w257]
          tunnel: u32[] [15790320, 15790320, 15790320, 15790320, 16777215, 16777215, 15790320, 15790320, 15790320] -> [_ _ _ _ w263]
          tunnel: w221 -> [_ _ _ _ w251]
          tunnel: w218 -> [_ w228 _ _ _]
          frame "Custom", Default {
          }
          frame "Basic" {
            n119 = call <vilib>:"WPI_DashboardUpdateNames.vi"("Controls on Tab"=w228) -> ()  [unwired: 11 in]
          }
          frame "Test" {
            w240 = -2 ("Active Item:Row Number")
            n120 = Index Array(array=w234, index=w233) -> (element=w235:T21)
            n121 = Unbundle(w235) -> ("Operation"=w236:enum16{"Update", "Clear"}, "Color Box"=w237:u32)
            n122 = call <vilib>:"NT Read String.vi"("Name"="/TestMode/TestName") -> ("String"=w231:string)  [unwired: 9 in, 1 out]
            n123 = call <vilib>:"NT Read and Format Entries as Tree.vi"("Operation"=w236, "Name Pattern"=w241, "Tree Refnum"=w242) -> ()  [unwired: 7 in, 2 out]
            n124 = case shown="\"\"" w231 {
              tunnel: "/TestMode/TestProgress" ("Name") -> [w244 _]
              tunnel: "/TestMode/TestProgressText" ("Name") -> [w243 _]
              frame Default {
                n125 = call <vilib>:"NT Read Number.vi"("Name"=w244) -> ("Numeric"=w245:dbl)  [unwired: 9 in, 1 out]
                n126 = call <vilib>:"NT Read String.vi"("Name"=w243) -> ("String"=w246:string)  [unwired: 9 in, 1 out]
                n127 = Bundle("Numeric"=w245, "String"=w246) -> (→"Progress":cluster{"Numeric":dbl, "String":string})  [unwired: 1 in]
              }
              frame "" {
                n128 = property on="Progress" class="Clust (strict)"("Visible"=FALSE) -> ()  [unwired: 2 in, 2 out]
                n129 = local write "Test Name"(u16 0) -> ()
              }
            }
            n130 = property on="Test Tree" class="Tree (strict)"("Active Item Row Number"=w240, "ActiveColNum"=w240, "CellBG"=w237, "Active Item Row Number"=-1 ("Active Item:Row Number"), "CellBG"=u32 5789784 ("Color Box")) -> ()  [unwired: 2 in, 2 out]
          }
          frame "Variables" {
            n131 = control-ref of="Tree"() -> (w250:refnum<vi>)
            n132 = call <vilib>:"NT Read and Format Entries as Tree.vi"("Tree Refnum"=w250) -> ()  [unwired: 9 in, 2 out]
          }
          frame "Commands" {
            w259 = u32 5789784 ("Color Box")
            w260 = T22 {"Row"=-1, "Column"=-2} ("Active Cell:Active Cell")
            w262 = T22 {"Row"=-2, "Column"=-2} ("Active Cell:Active Cell")
            n133 = Index Array(array=w263, index=w257) -> (element=w261:u32)
            n134 = Index Array(array=w258, index=w257) -> (element=w256:T21)
            n135 = Unbundle(w256) -> ("Operation"=w255:enum16{"Update", "Clear"})  [unwired: 1 out]
            n136 = local read "Command Selection"() -> (w254:i32)
            n137 = property on="Command Selection" class="MCListbox (strict)"("ActiveCell"=w262, "CellBG"=w261, "ActiveCell"=w260, "CellBG"=w259) -> ()  [unwired: 2 in, 2 out]
            n138 = call <vilib>:"WPI_DashboardUpdate RPC Info.vi"("Operation"=w255) -> ("update"=w253:bool, "commands"=w252:string[][])  [unwired: 9 in]
            n139 = property on="Command Selection" class="MCListbox (strict)"("ItemNames"=w252) -> ()  [unwired: 2 in, 2 out]
            n140 = property on="Command Params" class="Tbl (strict)"("Active Cell"=w262, "Cell BG Color"=w261, "Active Cell"=w260, "Cell BG Color"=w259) -> ()  [unwired: 2 in, 2 out]
            n141 = call <vilib>:"WPI_DashboardUpdate Command Params.vi"("Update"=w253, "NewVal"=w254, "Commands"=w252, "Param Tbl"=w251) -> ()  [unwired: 7 in, 1 out]
          }
        }
        n142 = call <vilib>:"Connextion Info.vi"() -> ("Connected"=→"NT Connection":bool)  [unwired: 10 in, 1 out]
      }
      event "Test Tree": Value Change {
        # "Show appropriate\ncontrols"
        n143 = event-data() -> ("CtlRef"=w268:refnum<vi>, "NewVal"=w266:string)  [unwired: 1 in]
        n144 = call <vilib>:"WPI_UtilitiesGetTreeIOName.vi"("NewVal"=w266, "TreeControl in"=w268) -> ("I/O Name"=w269:string)  [unwired: 9 in]
        n145 = case shown="\"Camera\"" w269 {
          selector: w269 -> [_ w276 _ w298 w307 _]
          tunnel: w266 -> [_ _ w295 w297 _ w314]
          tunnel: cluster{string[]}[] [{["640x480", "320x240", "160x120"]}, {["Auto", "Fixed indoor", "Fixed outdoor 1", "Fixed outdoor 2", "Fixed fluorescent 1", "Fixed fluorescent 2", "Hold current"]}, {["Auto", "Flicker-free 50 Hz", "Flicker-free 60 Hz", "Hold current"]}, {["None", "Prioritize frame rate", "Prioritize image quality"]}, {["Monochrome", "Color"]}] -> [_ _ _ _ _ w313]
          frame Default {
            w271 = FALSE ("Visible")
            w270 = FALSE ("Visible")
            n146 = property on="Motor" class="Clust (strict)"("Visible"=w270) -> ()  [unwired: 2 in, 2 out]
            n147 = property on="Test Ring" class="Ring (strict)"("Visible"=w270) -> ()  [unwired: 2 in, 2 out]
            n148 = property on="Rev/Fwd" class="Clust (strict)"("Visible"=w271) -> ()  [unwired: 2 in, 2 out]
            n149 = property on="On/Off" class="Bool (strict)"("Visible"=w271) -> ()  [unwired: 2 in, 2 out]
            n150 = property on="Test Slider" class="Slide (strict)"("Visible"=w271) -> ()  [unwired: 2 in, 2 out]
          }
          frame "Analog Out", "Motor", "PWM" {
            w277 = FALSE ("Visible")
            n151 = case shown="\"Analog Out\"" w276 {
              tunnel: [1.0 ("Value") -1.0 ("Value") 0.0 ("Value")] -> w275
              tunnel: [255.0 ("Value") 1.0 ("Value") 5.0 ("Value")] -> w274
              tunnel: [128.0 ("Value") 0.0 ("Value") 0.0 ("Value")] -> w273
              tunnel: [64.0 ("Value") 0.5 ("Value") 1.0 ("Value")] -> w272
              frame "PWM" {
              }
              frame "Motor", Default {
              }
              frame "Analog Out" {
              }
            }
            n152 = property on="Motor" class="Clust (strict)"("Visible"=TRUE) -> ()  [unwired: 2 in, 2 out]
            n153 = property on="Value" class="Slide (strict)"("Value"=w273, "Scale.Minimum"=w275, "Scale.Maximum"=w274, "Scale.Increment"=w272) -> ()  [unwired: 2 in, 2 out]
            n154 = property on="On/Off" class="Bool (strict)"("Visible"=w277) -> ()  [unwired: 2 in, 2 out]
            n155 = property on="Test Slider" class="Slide (strict)"("Visible"=w277) -> ()  [unwired: 2 in, 2 out]
            n156 = property on="Test Ring" class="Ring (strict)"("Visible"=w277) -> ()  [unwired: 2 in, 2 out]
            n157 = property on="Rev/Fwd" class="Clust (strict)"("Visible"=w277) -> ()  [unwired: 2 in, 2 out]
          }
          frame "Servo" {
            w293 = FALSE ("Visible")
            n158 = call <vilib>:"NT Read Number.vi"("Name"=w295) -> ("Numeric"=w294:dbl)  [unwired: 9 in, 1 out]
            n159 = property on="Test Slider" class="Slide (strict)"("Visible"=TRUE, "Scale.Maximum"=170.0 ("Scale.Range:Maximum")) -> ()  [unwired: 2 in, 2 out]
            n160 = local write "Test Slider"(w294) -> ()
            n161 = property on="Motor" class="Clust (strict)"("Visible"=w293) -> ()  [unwired: 2 in, 2 out]
            n162 = property on="Rev/Fwd" class="Clust (strict)"("Visible"=w293) -> ()  [unwired: 2 in, 2 out]
            n163 = property on="On/Off" class="Bool (strict)"("Visible"=w293) -> ()  [unwired: 2 in, 2 out]
            n164 = property on="Test Ring" class="Ring (strict)"("Visible"=w293) -> ()  [unwired: 2 in, 2 out]
          }
          frame "Relay", "Solenoid" {
            w296 = FALSE ("Visible")
            n165 = property on="Motor" class="Clust (strict)"("Visible"=w296) -> ()  [unwired: 2 in, 2 out]
            n166 = property on="Test Slider" class="Slide (strict)"("Visible"=w296) -> ()  [unwired: 2 in, 2 out]
            n167 = Search and Replace String(input string=w297, search string="/Value  **", replace string="/Direction") -> (result string=w303:string)  [unwired: 5 in, 3 out]
            n168 = property on="Test Ring" class="Ring (strict)"("Visible"=w296) -> ()  [unwired: 2 in, 2 out]
            n169 = call <vilib>:"NT Read String.vi"("Name"=w303) -> ("String"=w301:string)  [unwired: 9 in, 1 out]
            n170 = Equal?(x="Both directions", y=w301) -> (x = y?=w299:bool)
            n171 = Not(x=w299) -> (.not. x?=w300:bool)
            n172 = property on="Rev/Fwd" class="Clust (strict)"("Visible"=w299) -> ()  [unwired: 2 in, 2 out]
            n173 = property on="On/Off" class="Bool (strict)"("Visible"=w300, "Caption.Text"=w298) -> ()  [unwired: 2 in, 2 out]
          }
          frame "Compressor", "Digital Out" {
            w306 = FALSE ("Visible")
            # "Get direction and finish"
            n174 = property on="Motor" class="Clust (strict)"("Visible"=w306) -> ()  [unwired: 2 in, 2 out]
            n175 = property on="Test Slider" class="Slide (strict)"("Visible"=w306) -> ()  [unwired: 2 in, 2 out]
            n176 = property on="Test Ring" class="Ring (strict)"("Visible"=w306) -> ()  [unwired: 2 in, 2 out]
            n177 = property on="On/Off" class="Bool (strict)"("Visible"=TRUE, "Caption.Text"=w307) -> ()  [unwired: 2 in, 2 out]
            n178 = property on="Rev/Fwd" class="Clust (strict)"("Visible"=FALSE) -> ()  [unwired: 2 in, 2 out]
          }
          frame "Camera" {
            n179 = call <vilib>:"Get Last Path Segment.vi"("String in"=w314) -> ("String out"=w315:string)  [unwired: 10 in]
            n180 = property on="On/Off" class="Bool (strict)"("Visible"=FALSE) -> ()  [unwired: 2 in, 2 out]
            n181 = property on="Motor" class="Clust (strict)"("Visible"=FALSE) -> ()  [unwired: 2 in, 2 out]
            n182 = property on="Rev/Fwd" class="Clust (strict)"("Visible"=FALSE) -> ()  [unwired: 2 in, 2 out]
            n183 = case shown="\"White Balance  **\"" w315 {
              tunnel: w314 -> [w321 w330 w339 w348 w357 _ w363]
              tunnel: w313 -> [w319 w327 w336 w345 w354 _ _]
              frame "Size  **" {
                n184 = Index Array(array=w319) -> (element=w318:cluster{string[]})  [unwired: 1 in]
                n185 = call <vilib>:"NT Read String.vi"("Name"=w321) -> ("String"=w320:string)  [unwired: 9 in, 1 out]
                n186 = Unbundle(w318) -> (w316:string[])
                n187 = Match First String(2:w316, 3:w320) -> (0:w317:i32)  [unwired: 1 out]
                n188 = property on="Test Ring" class="Ring (strict)"("Value"=w317, "Strings []"=w316) -> ()  [unwired: 2 in, 2 out]
                n189 = property on="Test Ring" class="Ring (strict)"("Visible"=TRUE) -> ()  [unwired: 2 in, 2 out]
                n190 = property on="Test Slider" class="Slide (strict)"("Visible"=FALSE) -> ()  [unwired: 2 in, 2 out]
              }
              frame "White Balance  **" {
                n191 = Index Array(array=w327, index=1) -> (element=w328:cluster{string[]})
                n192 = call <vilib>:"NT Read String.vi"("Name"=w330) -> ("String"=w329:string)  [unwired: 9 in, 1 out]
                n193 = Unbundle(w328) -> (w325:string[])
                n194 = Match First String(2:w325, 3:w329) -> (0:w324:i32)  [unwired: 1 out]
                n195 = property on="Test Ring" class="Ring (strict)"("Value"=w324, "Strings []"=w325) -> ()  [unwired: 2 in, 2 out]
                n196 = property on="Test Ring" class="Ring (strict)"("Visible"=TRUE) -> ()  [unwired: 2 in, 2 out]
                n197 = property on="Test Slider" class="Slide (strict)"("Visible"=FALSE) -> ()  [unwired: 2 in, 2 out]
              }
              frame "Exposure  **" {
                n198 = Index Array(array=w336, index=2) -> (element=w337:cluster{string[]})
                n199 = call <vilib>:"NT Read String.vi"("Name"=w339) -> ("String"=w338:string)  [unwired: 9 in, 1 out]
                n200 = Unbundle(w337) -> (w333:string[])
                n201 = Match First String(2:w333, 3:w338) -> (0:w334:i32)  [unwired: 1 out]
                n202 = property on="Test Ring" class="Ring (strict)"("Value"=w334, "Strings []"=w333) -> ()  [unwired: 2 in, 2 out]
                n203 = property on="Test Ring" class="Ring (strict)"("Visible"=TRUE) -> ()  [unwired: 2 in, 2 out]
                n204 = property on="Test Slider" class="Slide (strict)"("Visible"=FALSE) -> ()  [unwired: 2 in, 2 out]
              }
              frame "Exposure Priority  **" {
                n205 = Index Array(array=w345, index=3) -> (element=w346:cluster{string[]})
                n206 = call <vilib>:"NT Read String.vi"("Name"=w348) -> ("String"=w347:string)  [unwired: 9 in, 1 out]
                n207 = Unbundle(w346) -> (w342:string[])
                n208 = Match First String(2:w342, 3:w347) -> (0:w343:i32)  [unwired: 1 out]
                n209 = property on="Test Ring" class="Ring (strict)"("Value"=w343, "Strings []"=w342) -> ()  [unwired: 2 in, 2 out]
                n210 = property on="Test Ring" class="Ring (strict)"("Visible"=TRUE) -> ()  [unwired: 2 in, 2 out]
                n211 = property on="Test Slider" class="Slide (strict)"("Visible"=FALSE) -> ()  [unwired: 2 in, 2 out]
              }
              frame "Color Enable  **" {
                n212 = Index Array(array=w354, index=4) -> (element=w355:cluster{string[]})
                n213 = call <vilib>:"NT Read String.vi"("Name"=w357) -> ("String"=w356:string)  [unwired: 9 in, 1 out]
                n214 = Unbundle(w355) -> (w351:string[])
                n215 = Match First String(2:w351, 3:w356) -> (0:w352:i32)  [unwired: 1 out]
                n216 = property on="Test Ring" class="Ring (strict)"("Value"=w352, "Strings []"=w351) -> ()  [unwired: 2 in, 2 out]
                n217 = property on="Test Ring" class="Ring (strict)"("Visible"=TRUE) -> ()  [unwired: 2 in, 2 out]
                n218 = property on="Test Slider" class="Slide (strict)"("Visible"=FALSE) -> ()  [unwired: 2 in, 2 out]
              }
              frame Default {
                n219 = property on="Test Ring" class="Ring (strict)"("Visible"=FALSE) -> ()  [unwired: 2 in, 2 out]
                n220 = property on="Test Slider" class="Slide (strict)"("Visible"=FALSE) -> ()  [unwired: 2 in, 2 out]
              }
              frame "Brightness  **", "Color Level  **", "Compression  **", "FPS  **", "Sharpness  **" {
                n221 = call <vilib>:"NT Read Number.vi"("Name"=w363) -> ("Numeric"=w362:dbl)  [unwired: 9 in, 1 out]
                n222 = local write "Test Slider"(w362) -> ()
                n223 = property on="Test Slider" class="Slide (strict)"("Visible"=TRUE, "Scale.Maximum"=100.0 ("Scale.Range:Maximum")) -> ()  [unwired: 2 in, 2 out]
                n224 = property on="Test Ring" class="Ring (strict)"("Visible"=FALSE) -> ()  [unwired: 2 in, 2 out]
              }
            }
          }
        }
        n225 = property on="Progress" class="Clust (strict)"("Visible"=FALSE) -> ()  [unwired: 2 in, 2 out]
      }
      event "Test Name": Mouse Enter {
        # "Populate the ring with the list of tests"
        n226 = event-data() -> ()  [unwired: 1 in, 1 out]
        n227 = call <vilib>:"NT Read String Array.vi"("Name"="/TestMode/TestList") -> ("String Array"=w371:string[])  [unwired: 9 in, 1 out]
        n228 = Build Array (concatenate)("Select the test to run...", w371) -> (w370:string[])
        n229 = property on="Test Name" class="Ring (strict)"("Strings []"=w370) -> ()  [unwired: 2 in, 2 out]
      }
      event "Test Name": Value Change {
        w373 = FALSE ("Visible")
        # "Tell the robot the test name to run"
        n230 = event-data() -> ("NewVal"=w377:u16)  [unwired: 1 in]
        n231 = property on="Test Name" class="Ring (strict)"() -> ("Strings []"=w378:string[])  [unwired: 2 in, 2 out]
        n232 = local write "Progress"(T6 {"Test Progress"=0, "Test Progress Text"=""} ("Progress")) -> ()
        n233 = Index Array(array=w378, index=w377) -> (element=w376:string)
        n234 = call <vilib>:"NT Write String.vi"("String"=w376, "Name"="/TestMode/TestName") -> ()  [unwired: 9 in, 1 out]
        n235 = property on="Progress" class="Clust (strict)"("Visible"=TRUE) -> ()  [unwired: 2 in, 2 out]
        n236 = property on="Motor" class="Clust (strict)"("Visible"=w373) -> ()  [unwired: 2 in, 2 out]
        n237 = property on="Test Slider" class="Slide (strict)"("Visible"=w373) -> ()  [unwired: 2 in, 2 out]
        n238 = property on="On/Off" class="Bool (strict)"("Visible"=w373) -> ()  [unwired: 2 in, 2 out]
        n239 = property on="Rev/Fwd" class="Clust (strict)"("Visible"=w373) -> ()  [unwired: 2 in, 2 out]
        n240 = property on="Test Ring" class="Ring (strict)"("Visible"=w373) -> ()  [unwired: 2 in, 2 out]
      }
      event "Select Auto": Mouse Enter {
        # "Populate the combo box with the list of autonomous options"
        n241 = event-data() -> ()  [unwired: 1 in, 1 out]
        n242 = call <vilib>:"NT Read String Array.vi"("Name"="Auto List") -> ("String Array"=w380:string[])  [unwired: 9 in, 1 out]
        n243 = property on="Select Auto" class="CmbBox"("Strings[]"=w380) -> ()  [unwired: 2 in, 2 out]
      }
      event "Select Auto": Value Change {
        # "User modified the Auto Selection. Write to NT variable so robot knows."
        n244 = event-data() -> ("NewVal"=w383:string)  [unwired: 1 in]
        n245 = call <vilib>:"NT Write String.vi"("String"=w383, "Name"="Auto Selector") -> ()  [unwired: 9 in, 1 out]
      }
      event "Command Selection": Value Change {
        # "Get the params and show in table"
        n246 = event-data() -> ("NewVal"=w389:i32)  [unwired: 1 in]
        n247 = property on="Command Selection" class="MCListbox (strict)"() -> ("ItemNames"=w387:string[][])  [unwired: 2 in, 2 out]
        n248 = call <vilib>:"WPI_DashboardUpdate Command Params.vi"("NewVal"=w389, "Commands"=w387, "Param Tbl"=w388) -> ()  [unwired: 8 in, 1 out]
      }
      event "Execute Command": Value Change {
        # "Started one, Unique ID holds\nresponse"
        n249 = event-data() -> ()  [unwired: 1 in, 1 out]
        n250 = property on="Command Selection" class="MCListbox (strict)"() -> ("ItemNames"=w400:string[][])  [unwired: 2 in, 2 out]
        n251 = Index Array(array=w400, index (row)="Command Selection", index (col)=0) -> (element=w398:string)
        n252 = call <vilib>:"Invoke Commands.vi"("Command Params"="Command Params", "Function Name"=w398) -> ("Params"=w394:u8, "Started"=w393:bool)  [unwired: 7 in, 1 out]
        n253 = Array Subset(array="Command Params", length (row)=w394) -> (w395:string[][])  [unwired: 3 in]
        n254 = Select(t="Executing" ("Cmd Status"), s=w393, f="" ("Cmd Status")) -> (s? t:f=→"Cmd Status":string)
      }
      event "Command Selection": Double Click {
        n255 = event-data() -> ("Row"=w408:i32)  [unwired: 1 in]
        n256 = property on="Command Selection" class="MCListbox (strict)"() -> ("ItemNames"=w411:string[][])  [unwired: 2 in, 2 out]
        n257 = local read "Command Params"() -> (w407:string[][])
        n258 = Index Array(array=w411, index (row)=w408, index (col)=0) -> (element=w409:string)
        n259 = call <vilib>:"Invoke Commands.vi"("Command Params"=w407, "Function Name"=w409) -> ("Params"=w406:u8, "Started"=w401:bool)  [unwired: 7 in, 1 out]
        n260 = Array Subset(array=w407, length (row)=w406) -> (w405:string[][])  [unwired: 3 in]
        n261 = Select(t="Executing" ("Cmd Status"), s=w401, f="" ("Cmd Status")) -> (s? t:f=w402:string)
        n262 = local write "Cmd Status"(w402) -> ()
      }
      event "CheckList": Double Click {
        # "Shift clears all"
        # "Update symbols on the listbox"
        n263 = event-data() -> ("PlatMods.Shift"=w413:bool, "Row"=w415:i32)  [unwired: 1 in]
        n264 = case shown="True" w413 {
          tunnel: w415 -> [w419 _]
          tunnel: 1 -> [w418 _]
          frame False {
            n265 = property on="CheckList" class="LstBox (strict)"() -> ("Item Symbols"=w417:i32[])  [unwired: 2 in, 2 out]
            n266 = Replace Array Subset(array=w417, new element=w418, index=w419) -> (w416:i32[])
            n267 = property on="CheckList" class="LstBox (strict)"("Item Symbols"=w416) -> ()  [unwired: 2 in, 2 out]
          }
          frame True {
            w420 = 0 ("Top Row")
            n268 = property on="CheckList" class="LstBox (strict)"() -> ("Number of Rows"=w422:u32)  [unwired: 2 in, 2 out]
            n269 = Initialize Array(0, w422) -> (w421:i32[])
            n270 = property on="CheckList" class="LstBox (strict)"("Top Row"=w420, "Value"=w420, "Item Symbols"=w421) -> ()  [unwired: 2 in, 2 out]
          }
        }
      }
      event "CheckList": Key Down {
        # "Update symbols on the listbox\nLeft and right keys check and uncheck"
        n271 = event-data() -> ("VKey"=w426:T19)  [unwired: 1 in]
        n272 = case shown="\"Left\", \"Right\"" w426 {
          selector: w426 -> [w431 _]
          tunnel: eventvkey."Left" ("VKey") -> [w429 _]
          frame "Left", "Right" {
            n273 = Equal?(x=w429, y=w431) -> (x = y?=w430:bool)
            n274 = Select(t=0, s=w430, f=1) -> (s? t:f=w432:i32)
            n275 = property on="CheckList" class="LstBox (strict)"() -> ("Item Symbols"=w435:i32[])  [unwired: 2 in, 2 out]
            n276 = Replace Array Subset(array=w435, new element=w432, index="CheckList") -> (w434:i32[])
            n277 = property on="CheckList" class="LstBox (strict)"("Item Symbols"=w434) -> ()  [unwired: 2 in, 2 out]
          }
          frame Default {
          }
        }
      }
      event "Motor.Enable": Value Change {
        # "When the test mode otor enable helper is set, update that\ntree row item's value"
        n278 = event-data() -> ("NewVal"=w441:bool)  [unwired: 1 in]
        n279 = Unbundle("Motor") -> ("Value"=w440:dbl)  [unwired: 1 out]
        n280 = Select(t=w440, s=w441, f=0.0) -> (s? t:f=w438:dbl)
        n281 = call <vilib>:"NT Write Number.vi"("Numeric"=w438, "Name"=w437) -> ()  [unwired: 9 in, 1 out]
      }
      event "Test Slider": Value Change {
        # "When the test mode slider helper is set, update that\ntree row item's value"
        n282 = event-data() -> ("NewVal"=w444:dbl)  [unwired: 1 in]
        n283 = call <vilib>:"NT Write Number.vi"("Numeric"=w444, "Name"=w445) -> ()  [unwired: 9 in, 1 out]
      }
      event "On/Off": Value Change {
        # "When the test mode on/off helper value is set, update that\ntree row item's value"
        n284 = event-data() -> ("NewVal"=w449:bool)  [unwired: 1 in]
        n285 = Boolean To (0,1)(Boolean=w449) -> (0, 1=w448:i16)
        n286 = call <vilib>:"NT Write Number.vi"("Numeric"=w448, "Name"=w447) -> ()  [unwired: 9 in, 1 out]
      }
      event "Rev/Fwd": Value Change {
        # "When the test mode helper value for relays is set, update that\ntree row item's value"
        n287 = event-data() -> ("NewVal.Forward"=w457:bool, "NewVal.Reverse"=w456:bool)  [unwired: 1 in]
        n288 = Boolean To (0,1)(Boolean=w457) -> (0, 1=w453:i16)
        n289 = Boolean To (0,1)(Boolean=w456) -> (0, 1=w455:i16)
        n290 = Negate(x=w455) -> (-x=w454:i16)
        n291 = Add(x=w453, y=w454) -> (x+y=w452:i16)
        n292 = call <vilib>:"NT Write Number.vi"("Numeric"=w452, "Name"=w451) -> ()  [unwired: 9 in, 1 out]
      }
      event "Test Ring": Value Change {
        # "When a test mode helper value is selected from the ring,\nset the tree item's variable to the string value"
        n293 = event-data() -> ("NewVal"=w461:u16)  [unwired: 1 in]
        n294 = property on="Test Ring" class="Ring (strict)"() -> ("Strings []"=w462:string[])  [unwired: 2 in, 2 out]
        n295 = Index Array(array=w462, index=w461) -> (element=w460:string)
        n296 = call <vilib>:"NT Write String.vi"("String"=w460, "Name"=w459) -> ()  [unwired: 9 in, 1 out]
      }
      event "Rec Mode": Value Change {
        # "Update globals for recording mode and path to read log from.\nClear when logging and let NetworkTables set path for vision to\nuse."
        n297 = event-data() -> ("NewVal"=w473:enum32{"Stop", "Record", "Playback"})  [unwired: 1 in]
        n298 = global write "WPI_DashboardLogging Global.vi" "Logging Filename"(path "") -> ()
        n299 = global write "WPI_DashboardLogging Global.vi" "Recording"(w473) -> ()
        n300 = case shown="\"Playback\"" w473 {
          tunnel: w472 -> [_ w475 w484]
          tunnel: [_ _ w483] -> w470
          tunnel: [_ _ w482] -> _
          tunnel: w468 -> [_ _ w480]
          tunnel: cluster{i32, i32} {-250, 170} -> [_ _ w479]
          tunnel: [_ _ T20 {"Image Size"=TRUE, "Image Type"=TRUE, "Pixel Value"=TRUE, "ROI Information"=TRUE, "Zoom Factor"=FALSE} ("Image Information Shown:All Elements")] -> w466
          tunnel: [_ _ TRUE ("Zoom Factor")] -> w465
          tunnel: w464 -> [_ _ w476]
          frame Default {
          }
          frame "Stop", "Record" {
            # "Place Window too"
            n301 = invoke class="VI" method="FP.Close"(reference=w475) -> (reference out=w474:refnum<vi>)  [unwired: 2 in, 2 out]
            n302 = invoke class="VI" method="Abort VI"(reference=w474) -> ()  [unwired: 2 in, 3 out]
          }
          frame "Playback" {
            n303 = call "Open Playback Panel.vi"("Offset"=w479, "DB VI Ref"=w480, "Playback in"=w484) -> ("Playback out"=w481:refnum<vi>)  [unwired: 8 in]
            n304 = register-events(w481, w476) -> (reference out=w483:refnum<event-registration>, error out=w482:errorcluster)  [unwired: 2 in]
          }
        }
        n305 = property on="Camera Image" class="ImageControl"("Image Information Shown"=w466, "Image Information Visible"=w465) -> ()  [unwired: 2 in, 2 out]
        n306 = call <vilib>:"WPI_DashboardNT Log FieldName Cache.vi"("Operation"=enum16{"Lookup/Add", "Index", "Clear"}."Clear") -> ()  [unwired: 8 in, 3 out]
      }
      event Panel Close {
        w486 = enum32{"Stop", "Record", "Playback"}."Stop" ("Rec Mode")
        # "Playback window has been closed, abort"
        n307 = event-data() -> ()  [unwired: 1 in, 4 out]
        n308 = local write "Rec Mode"(w486) -> ()
        n309 = global write "WPI_DashboardLogging Global.vi" "Recording"(w486) -> ()
      }
      event Panel Close {
        # "Abort playback window and ourself"
        n310 = event-data() -> ()  [unwired: 1 in, 4 out]
        n311 = invoke class="VI" method="FP.Close"(reference=w490) -> (reference out=w489:refnum<vi>)  [unwired: 2 in, 2 out]
        n312 = invoke class="VI" method="Abort VI"(reference=w489) -> (error out=w488:errorcluster)  [unwired: 2 in, 2 out]
        n313 = invoke class="VI" method="Abort VI"(error in=w488) -> ()  [unwired: 2 in, 3 out]
      }
      event User Event {
        n314 = event-data() -> ("IDs"=w497:cluster{"RPC field ID":u16, "Unique ID":u16}, "String"=w496:string)  [unwired: 1 in]
        n315 = Bundle("IDs"=w497, "String"=w496) -> (w495:T8)  [unwired: 1 in]
        n316 = call <vilib>:"Retrieve RPC Response.vi"("RPC Response"=w495) -> ("Output"=w493:string[][])  [unwired: 10 in]
        n317 = Build Array (concatenate)(w491, w493) -> (w492:string[][])
        n318 = local write "Command Params"(w492) -> ()
        n319 = local write "Cmd Status"("" ("Cmd Status")) -> ()
      }
      event "Tree": Double Click {
        n320 = event-data() -> ("PlatMods"=w501:T23, "Tag"=w500:string)  [unwired: 1 in]
        n321 = Unbundle(w501) -> ("Shift"=w499:bool)  [unwired: 4 out]
        n322 = Not(x=w499) -> (.not. x?=w498:bool)
        n323 = call <vilib>:"NT Update Persistence.vi"("Persistence"=w498, "Name"=w500) -> ()  [unwired: 9 in, 1 out]
      }
    }
  }
  n324 = while {
    tunnel: w64 -> [w504]
    i -> [w507]
    stop <- FALSE stop-if-true
    n325 = Wait (ms)(milliseconds to wait=u32 100) -> ()  [unwired: 1 out]
    n326 = case shown="\"Playback\"" "Rec Mode" {
      tunnel: w507 -> [_ _ w522]
      tunnel: [u32 2829099 ("Base Color") u32 11141120 ("Target Color") w511] -> w503
      frame "Stop", Default {
        # "Reset the color, extra updates don't cost much"
      }
      frame "Record" {
      }
      frame "Playback" {
        # "Playback"
        n327 = Quotient & Remainder(x=w522, y=u32 50 ("milliseconds to wait")) -> (x-y*floor(x/y)=w518:u32)  [unwired: 1 out]
        n328 = Divide(x=w518, y=u32 50 ("milliseconds to wait")) -> (x/y=w515:dbl)
        n329 = Multiply(x=6.283185307179586, y=w515) -> (x*y=w520:dbl)
        n330 = Sine(x=w520) -> (sin(x)=w519:dbl)
        n331 = Absolute Value(x=w519) -> (abs(x)=w512:dbl)
        n332 = call "Interpolate RGB Color.vi"("Proportion"=w512, "Target Color"=u32 30976, "Base Color"=u32 2829099) -> ("Result Color"=w511:u32)  [unwired: 8 in]
      }
    }
    n333 = property class="Pane"(reference=w504, "PaneColor"=w503) -> ()  [unwired: 1 in, 2 out]
  }
  n334 = local write "Dashboard Tab"(T2."Drive" ("Dashboard Tab")) -> ()
  n335 = property on="On/Off" class="Bool (strict)"("Visible"=w33) -> ()  [unwired: 2 in, 2 out]
  n336 = property on="Motor" class="Clust (strict)"("Visible"=w33) -> ()  [unwired: 2 in, 2 out]
  n337 = property on="Progress" class="Clust (strict)"("Visible"=w33) -> ()  [unwired: 2 in, 2 out]
  n338 = property on="Test Ring" class="Ring (strict)"("Visible"=w33) -> ()  [unwired: 2 in, 2 out]
  n339 = property on="Rev/Fwd" class="Clust (strict)"("Visible"=w33) -> ()  [unwired: 2 in, 2 out]
  n340 = local write "Command Selection"(u16 0 ("milliseconds to wait")) -> ()
  n341 = local write "Command Params"(string[][] [] ("Command Params")) -> ()
  n342 = global write "WPI_DashboardLogging Global.vi" "Recording"(w58) -> ()
  n343 = local write "Rec Mode"(w58) -> ()
  n344 = while {
    tunnel: u16 1741 ("timeout ms (25000)") -> [w524]
    stop <- FALSE stop-if-true
    n345 = TCP Create Listener(10:w524) -> (0:w523:errorcluster, 3:w525:refnum<k5>)  [unwired: 4 in, 1 out]
    n346 = case shown="No Error" w523 {
      selector: w523 -> [w527 _]
      tunnel: w525 -> [w528 _]
      frame No Error {
        n347 = while {
          tunnel: w528 -> [w531]
          tunnel: w527 -> [w530]
          stop <- FALSE stop-if-true
          n348 = TCP Wait On Listener(8:w530, 11:w531) -> (0:w532:errorcluster, 4:w533:refnum<k5>)  [unwired: 2 in, 3 out]
          n349 = local write "TCP"(w533) -> ()
          n350 = case shown="No Error" w532 {
            frame No Error {
            }
            frame Error {
              n351 = Wait (ms)(milliseconds to wait=u32 1000) -> ()  [unwired: 1 out]
            }
          }
        }
      }
      frame Error {
        n352 = Wait (ms)(milliseconds to wait=u32 1000) -> ()  [unwired: 1 out]
      }
    }
  }
  n353 = call <vilib>:"NT Write String.vi"("String"="Select Auto", "Name"="Auto Selector") -> ()  [unwired: 9 in, 1 out]
